vi "Process.vi"(8 "error in":errorcluster, 11 "Instrument.Aerotech":refnum<class "Instrument.Aerotech.lvclass">) -> (0 "error out":errorcluster, 3 "Instrument.Aerotech out":refnum<class "Instrument.Aerotech.lvclass">)   [LabVIEW 2019, in "Instrument.Aerotech.lvclass"]
doc: "---------------------------------------------------------------\nJKI State Machine Objects™\nhttp://jki.net/state-machine-objects/\nCopyright (C) 2005-2015, JKI <info@jki.net>\nALL RIGHTS RESERVED"
uses:
  Instrument.Aerotech.lvclass
  <vilib>/JKI/JKI SMO/SMO/SMO.lvclass
  <vilib>/JKI/JKI SMO/SMO/Typedefs/Parent Call--Enum.ctl
  C:/Program Files (x86)/National Instruments/LabVIEW 2019/user.lib/LevyLab/Instrument Framework/Instrument Types/Delay Line/Instrument.DelayLine.lvclass
  C:/Program Files (x86)/National Instruments/LabVIEW 2019/user.lib/LevyLab/Instrument Framework/Instrument/Instrument.lvclass
  C:/Program Files (x86)/National Instruments/LabVIEW 2019/vi.lib/JKI/JKI SMO/SMO/SMO.lvclass
  <userlib>/LevyLab/Instrument Framework/Instrument Types/Delay Line/Instrument.DelayLine.lvclass
panel:
  # "Example INSTRUMENT"
  # "For instructions on how to use the JKI State Machine Objects, examples and video tutorials, visit:\nhttp://jki.net/state-machine-objects/\n\nJKI State Machine Objects™\nhttp://jki.net/state-machine-objects/\nCopyright (C) 2005-2015, JKI <info@jki.net>\nALL RIGHTS RESERVED"
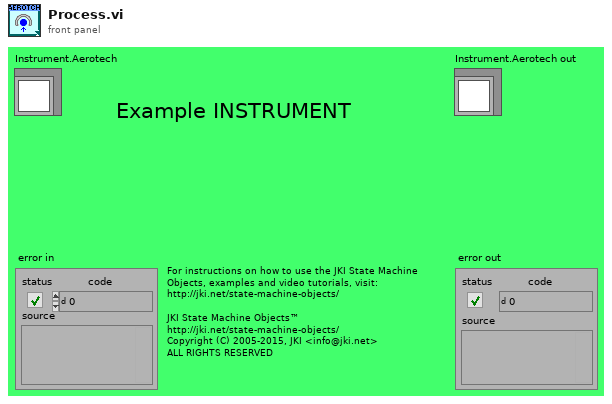
[diagram p1: front panel]
types:
  T1 = typedef "SMO.lvclass/Parent Call--Enum.ctl" = enum16{"Allows parent to run", "Does not request parent to run"}
  T2 = enum32{"invalid app kind", "Development System", "Run Time System", "Student Edition", "Embedded LabVIEW", "Evaluation", "Custom"}
  T3 = enum32{"Invalid", "Standard", "Closed", "Hidden", "Minimized", "Maximized"}
  T4 = enum32{"Bad", "Idle", "Run top level", "Running"}
  T5 = cluster{"Core":cluster{"Current VI Reference":refnum<vi>, "Close Panel on Exit?":bool, "error":errorcluster}, "Self Reference":refnum<class "Instrument.Aerotech.lvclass">}
  T6 = cluster{"Current VI Reference":refnum<vi>, "Close Panel on Exit?":bool, "error":errorcluster}
  T7 = typedef "SMO.lvclass/Protected Events.ctl" = cluster{"StopProcesses":refnum<user-event>, "AbortProcesses":refnum<user-event>, "Config Changed":refnum<user-event>, "Dependency":refnum<user-event>}
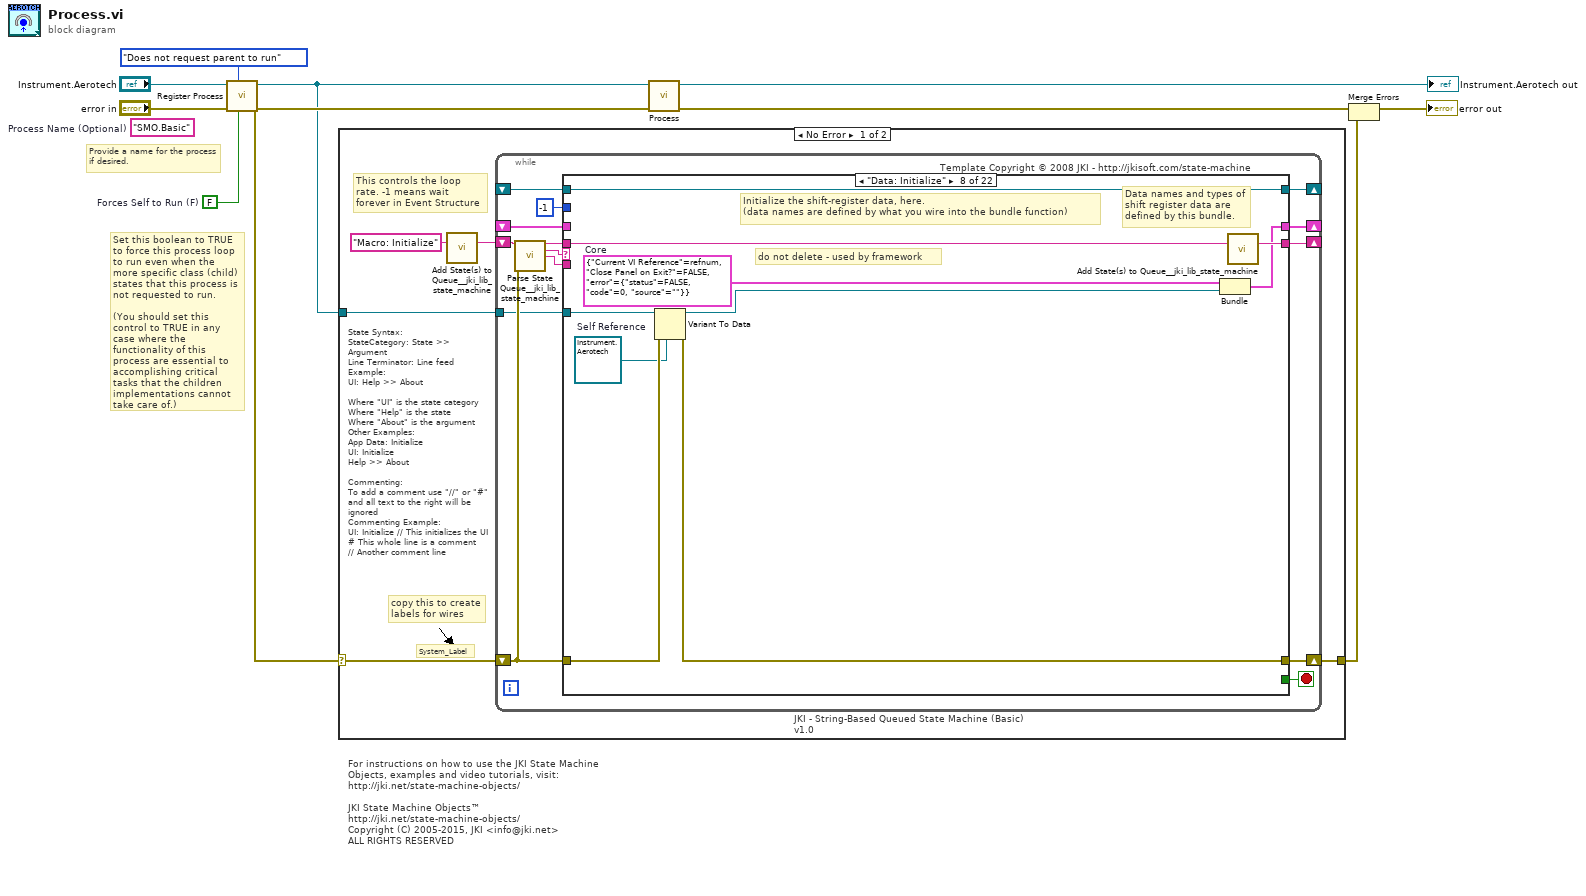
[diagram p0: block diagram]
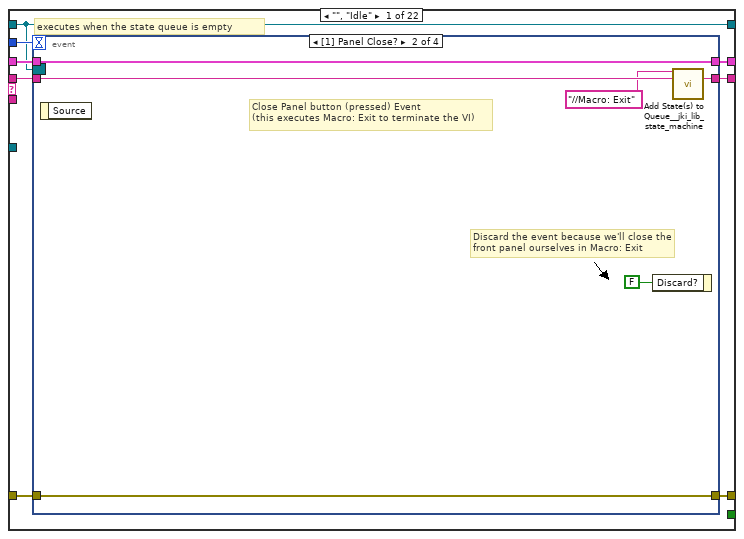
[diagram p2: hidden frame]
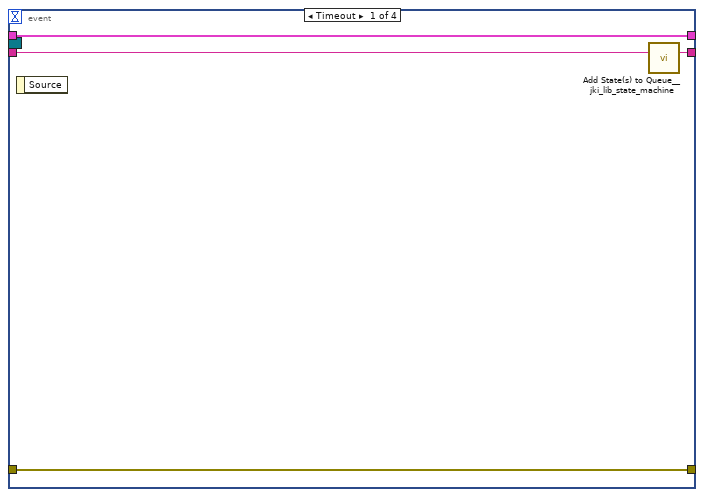
[diagram p3: hidden frame]
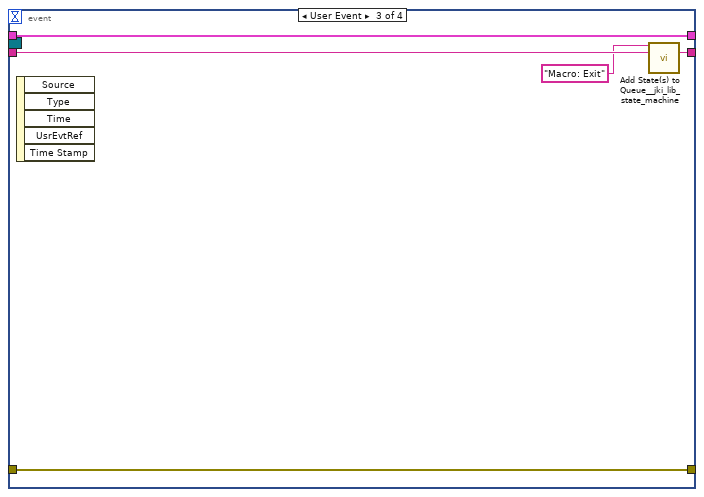
[diagram p4: hidden frame]
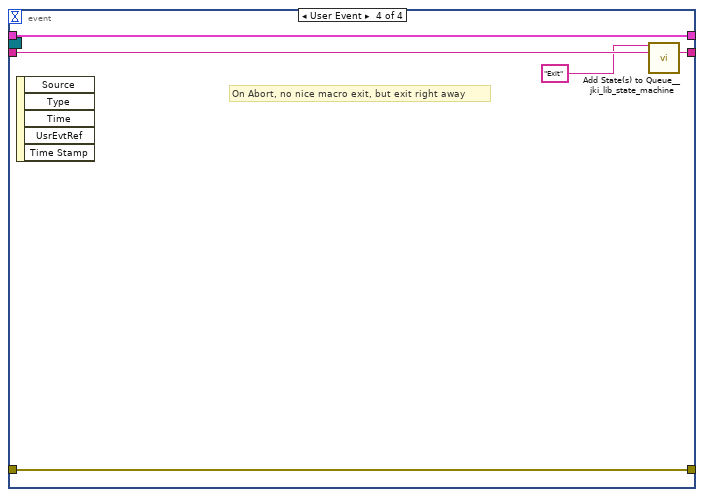
[diagram p5: hidden frame]
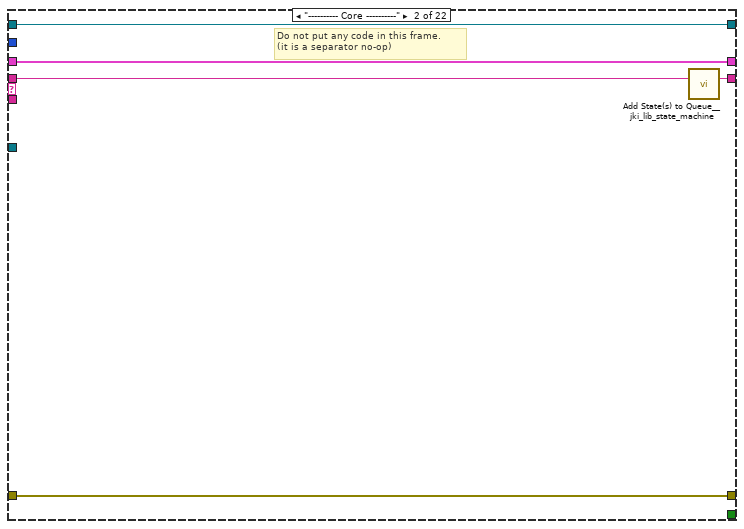
[diagram p6: hidden frame]
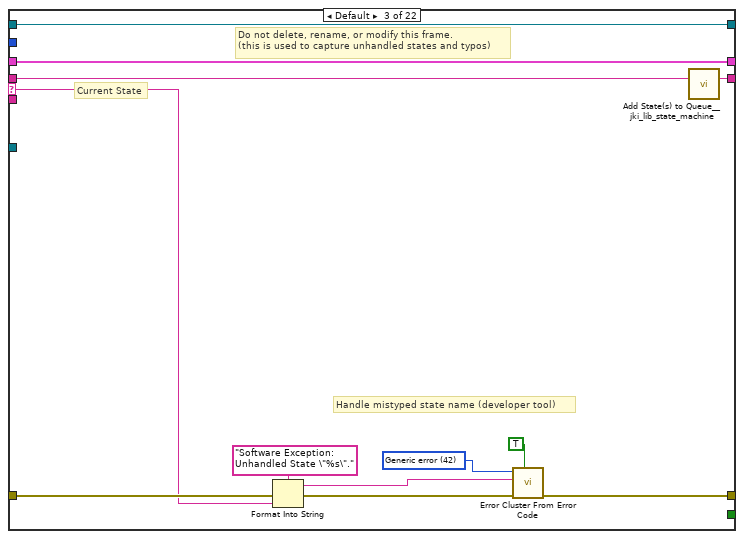
[diagram p7: hidden frame]
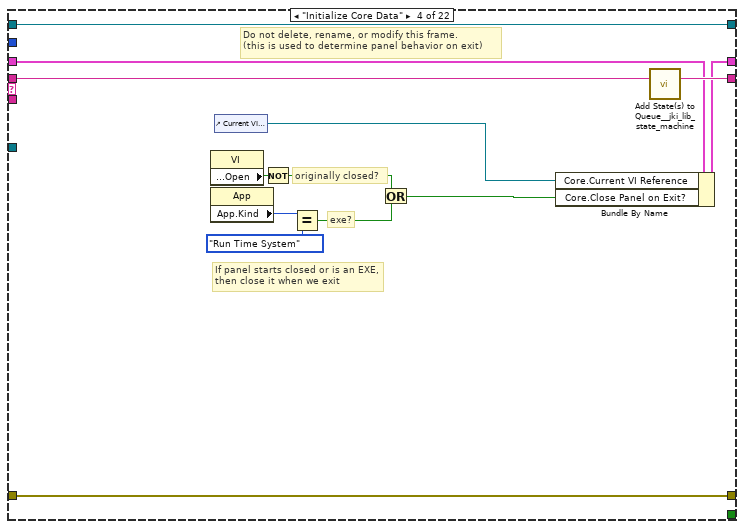
[diagram p8: hidden frame]
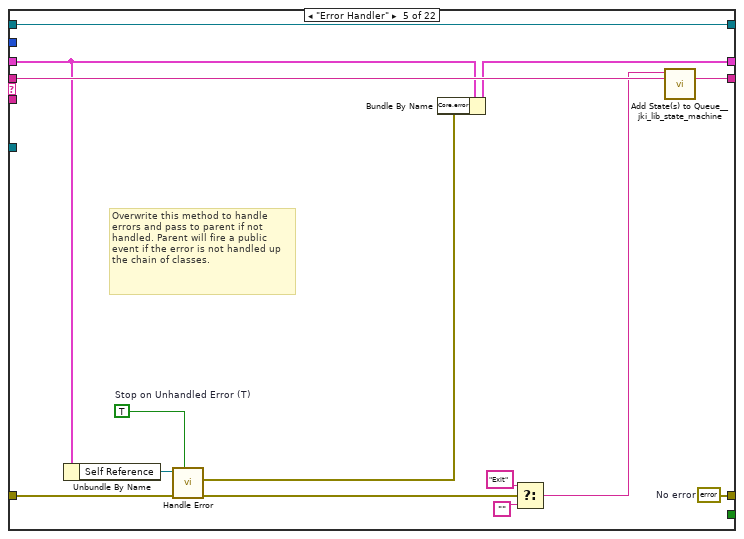
[diagram p9: hidden frame]
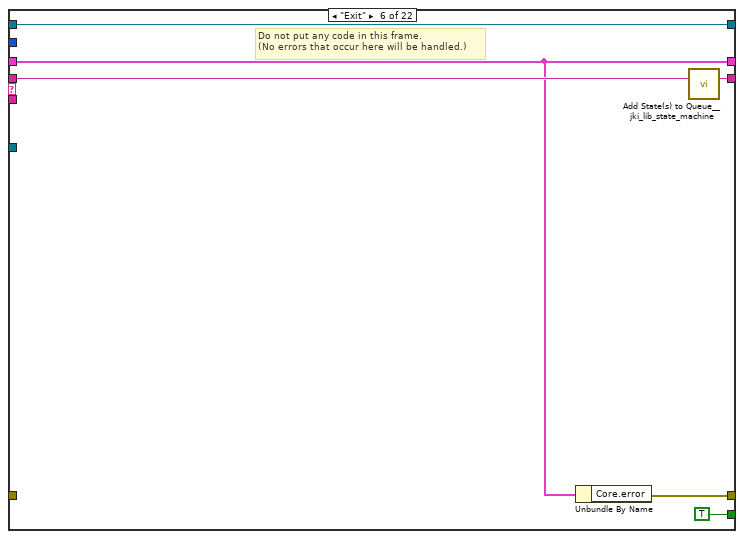
[diagram p10: hidden frame]
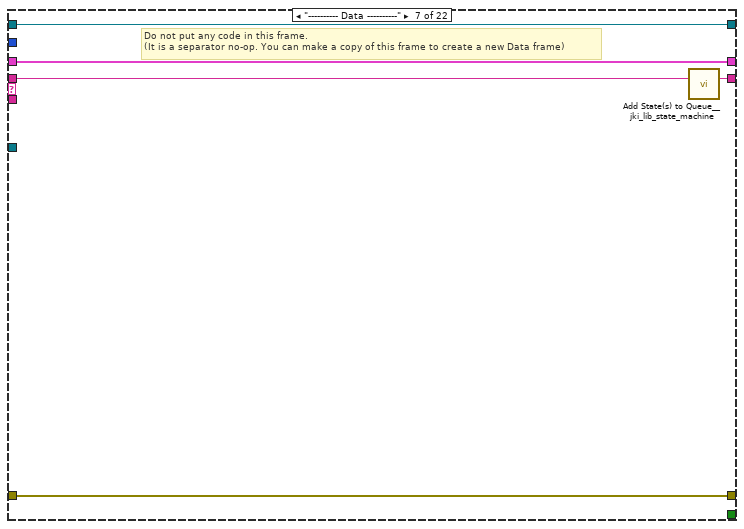
[diagram p11: hidden frame]
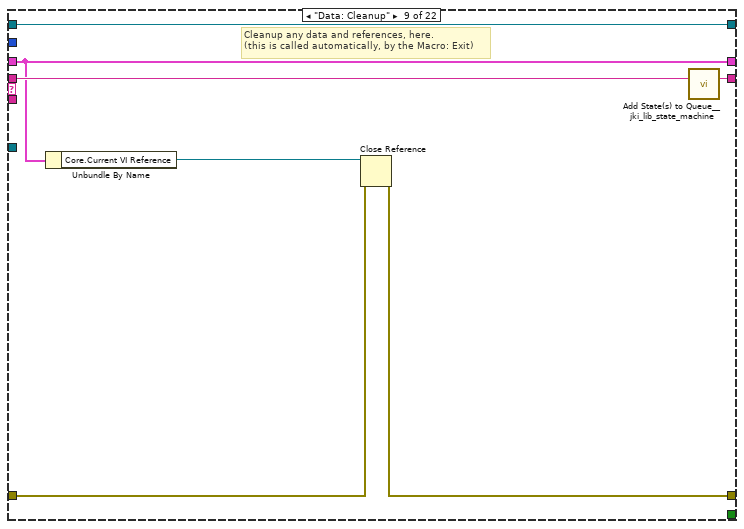
[diagram p12: hidden frame]
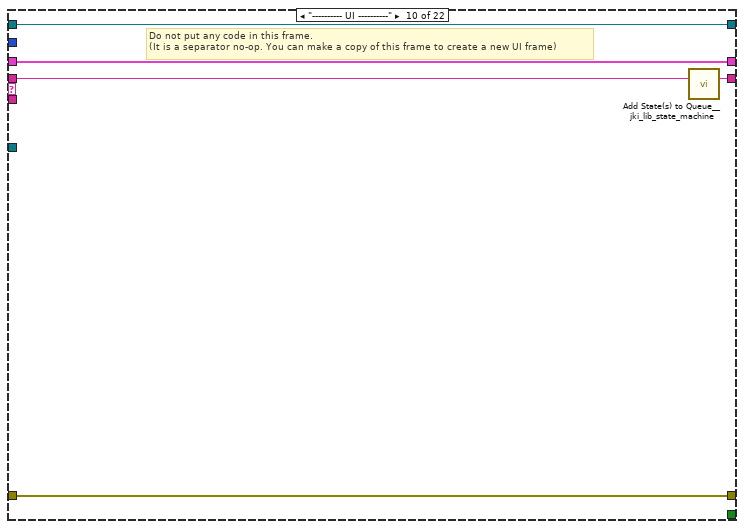
[diagram p13: hidden frame]
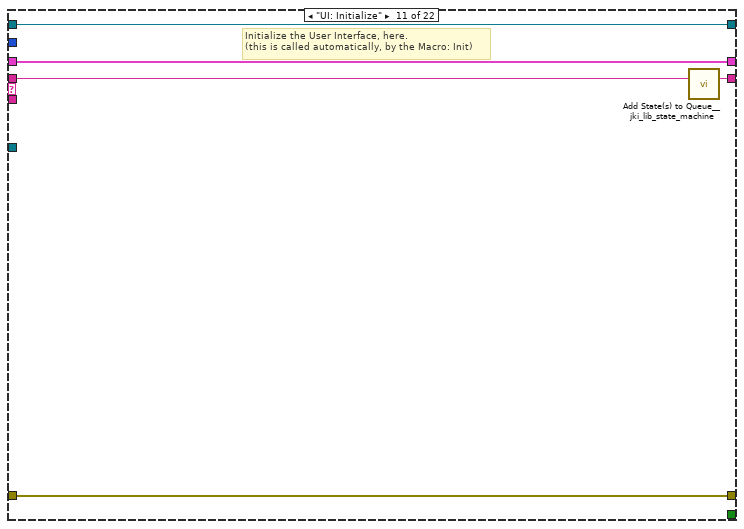
[diagram p14: hidden frame]
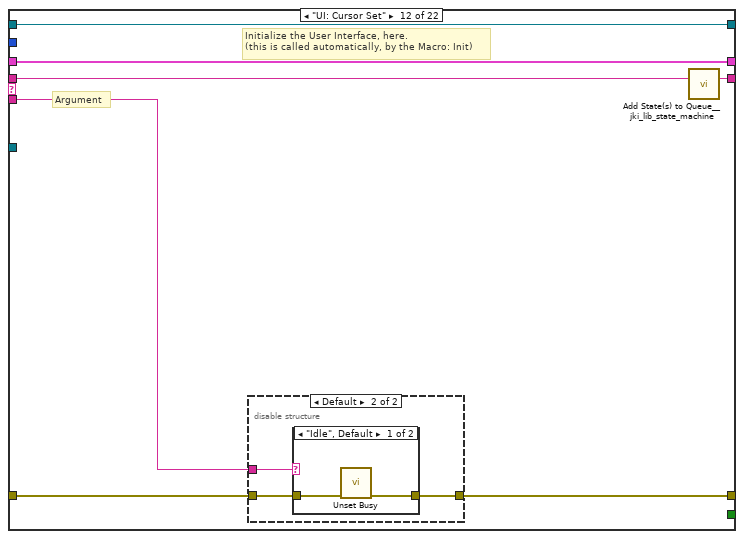
[diagram p15: hidden frame]
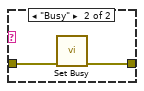
[diagram p17: hidden frame]
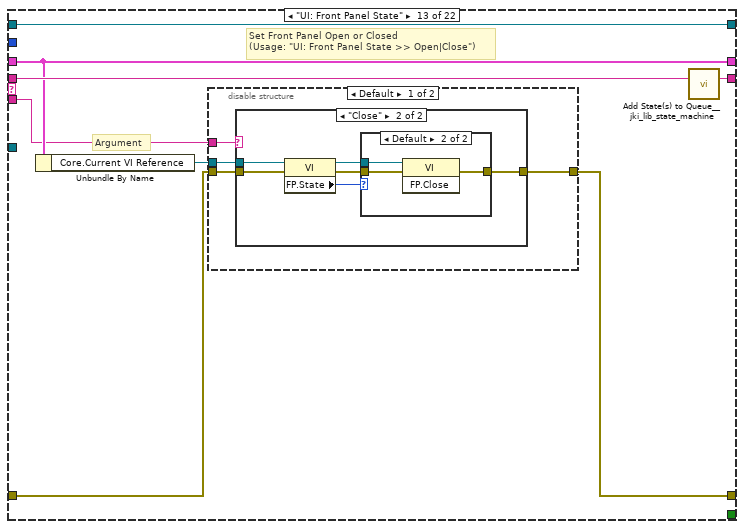
[diagram p18: hidden frame]
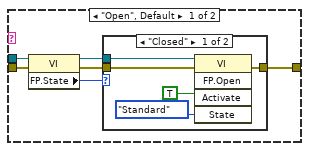
[diagram p19: hidden frame]
diagram:
  w1 = FALSE  # Forces Self to Run (F)
  (unwired) "SMO.Basic"  # Process Name (Optional)
  # "Provide a name for the process\nif desired."
  # "Set this boolean to TRUE to force this process loop to run even when the more specific class (child) states that this process is not requested to run.\n\n(You should set this control to TRUE in any case where the functionality of this process are essential to accomplishing critical tasks that the children implementations cannot take care of.)"
  # "For instructions on how to use the JKI State Machine Objects, examples and video tutorials, visit:\nhttp://jki.net/state-machine-objects/\n\nJKI State Machine Objects™\nhttp://jki.net/state-machine-objects/\nCopyright (C) 2005-2015, JKI <info@jki.net>\nALL RIGHTS RESERVED"
  n1 = call <vilib>:"Register Process.vi"("Forces Self to Run (F)"=w1, "Parent Call"=Parent_Call--Enum."Does not request parent to run", "error in (no error)"="error in", "SMO"="Instrument.Aerotech") -> ("error out"=w7:errorcluster, "SMO out"=w6:refnum<class "Instrument.Aerotech.lvclass">)  [unwired: 6 in]
  n2 = case shown="No Error" w7 {
    selector: w7 -> [w12 w265]
    tunnel: w6 -> [w13 _]
    tunnel: [w11 w265] -> w3
    frame No Error {
      # "State Syntax:\nStateCategory: State >> Argument\nLine Terminator: Line feed\nExample:\nUI: Help >> About\n\nWhere \"UI\" is the state category\nWhere \"Help\" is the state\nWhere \"About\" is the argument\nOther Examples:\nApp Data: Initialize\nUI: Initialize\nHelp >> About\n\nCommenting:\nTo add a comment use \"//\" or \"#\" and all text to the right will be ignored\nCommenting Example:\nUI: Initialize // This initializes the UI\n# This whole line is a comment\n// Another comment line"
      # "copy this to create labels for wires"
      # "This controls the loop rate. -1 means wait forever in Event Structure"
      # "System_Label"
      n3 = call <vilib>:"Add State(s) to Queue__jki_lib_state_machine.vi"("State(s) in (\"\")"="Macro: Initialize") -> ("States Out"=w15:string)  [unwired: 14 in]
      n4 = while "JKI - String-Based Queued State Machine (Basic) v1.0" {
        shift-right: [w22] -> _
        shift-left: _ -> [w21]
        shift-right: [w25] -> w11
        shift-left: w12 -> [w19]
        shift-right: [w24] -> _
        shift-left: w15 -> [w26]
        tunnel: w13 -> [w18]
        shift-right: [w17] -> _
        shift-left: _ -> [w16]
        stop <- w23 stop-if-true
        # "Template Copyright © 2008 JKI - http://jkisoft.com/state-machine"
        n5 = call <vilib>:"Parse State Queue__jki_lib_state_machine.vi"("State Queue"=w26, "Error In (no error)"=w19) -> ("Remaining States"=w28:string, "Current State"=w29:string, "Arguments"=w27:string)  [unwired: 11 in]
        n6 = case shown="\"Data: Initialize\"" w29 {
          selector: w29 -> [_ _ w64 _ _ _ _ _ _ _ _ _ _ _ _ _ _ _ _ _ _ _]
          tunnel: w28 -> [w37 w62 w68 w87 w101 w107 w112 w122 w129 w134 w139 w146 w162 w194 w208 w222 w227 w238 w243 w253 w259 w264]
          tunnel: w27 -> [_ _ _ _ _ _ _ _ _ _ _ w140 w156 _ _ _ _ _ _ _ _ _]
          tunnel: w21 -> [w35 w59 w66 w78 w95 w103 w109 _ w124 w131 w137 w144 w158 w191 w204 w213 w224 w235 w240 w244 w257 w262]
          tunnel: [w34 w60 w70 w84 w96 w102 w110 w118 w125 w132 w136 w141 w159 w192 w206 w220 w225 w229 w241 w248 w255 w260] -> w25
          tunnel: w19 -> [w33 w60 w69 w84 w97 _ w110 w119 w126 w132 w136 w142 w160 w192 w206 w220 w225 w230 w241 w249 w255 w260]
          tunnel: [w36 w61 w67 w86 w100 w106 w111 w121 w128 w133 w138 w145 w161 w193 w207 w221 w226 w237 w242 w252 w258 w263] -> w24
          tunnel: [_ _ _ _ _ TRUE _ _ _ _ _ _ _ _ _ _ _ _ _ _ _ _] -> w23
          tunnel: [w32 w59 w66 w85 w94 w103 w109 w120 w124 w131 w137 w144 w158 w191 w204 w213 w224 w235 w240 w244 w257 w262] -> w22
          tunnel: -1 ("Timeout") -> [w31 _ _ _ _ _ _ _ _ _ _ _ _ _ _ _ _ _ _ _ _ _]
          tunnel: w18 -> [_ _ _ _ _ _ _ w116 _ _ _ _ _ _ _ _ _ _ _ _ _ _]
          tunnel: [w30 w58 w63 w75 w99 w104 w108 w115 w123 w130 w135 w143 w155 w190 w205 w214 w223 w236 w239 w251 w256 w261] -> w17
          tunnel: w16 -> [w30 w58 w63 w75 w99 w104 w108 w115 w123 w130 w135 w143 w155 w190 w205 w214 w223 w236 w239 _ w256 w261]
          frame "", "Idle" {
            # "executes when the state queue is empty"
            n7 = event shown="[1] Panel Close?" {
              selector: w30 -> [_ _ _ _]
              dyn-events: _ -> [_ _ _ _]
              timeout: w31 -> [_ _ _ _]
              tunnel: w37 -> [w41 w47 w52 w57]
              tunnel: [w40 w46 w51 w56] -> w36
              tunnel: w35 -> [w38 w44 w49 w54]
              tunnel: [w39 w45 w50 w55] -> w34
              tunnel: w33 -> [w39 w45 w50 w55]
              tunnel: [w38 w44 w49 w54] -> w32
              event Timeout {
                n8 = event-data() -> ()  [unwired: 1 in, 1 out]
                n9 = call <vilib>:"Add State(s) to Queue__jki_lib_state_machine.vi"("State(s) in (\"\")"=w41) -> ("States Out"=w40:string)  [unwired: 14 in]
              }
              event Panel Close? {
                # "Discard the event because we'll close the front panel ourselves in Macro: Exit"
                # "Close Panel button (pressed) Event\n(this executes Macro: Exit to terminate the VI)"
                n10 = event-data() -> ()  [unwired: 1 in, 1 out]
                n11 = event-data("Discard?"=FALSE) -> ()  [unwired: 1 in, 1 out]
                n12 = call <vilib>:"Add State(s) to Queue__jki_lib_state_machine.vi"("State(s) in Front (\"\")"="//Macro: Exit", "State(s) in (\"\")"=w47) -> ("States Out"=w46:string)  [unwired: 13 in]
              }
              event User Event {
                n13 = event-data() -> ()  [unwired: 1 in, 5 out]
                n14 = call <vilib>:"Add State(s) to Queue__jki_lib_state_machine.vi"("State(s) in Front (\"\")"="Macro: Exit", "State(s) in (\"\")"=w52) -> ("States Out"=w51:string)  [unwired: 13 in]
              }
              event User Event {
                # "On Abort, no nice macro exit, but exit right away"
                n15 = event-data() -> ()  [unwired: 1 in, 5 out]
                n16 = call <vilib>:"Add State(s) to Queue__jki_lib_state_machine.vi"("State(s) in Front (\"\")"="Exit", "State(s) in (\"\")"=w57) -> ("States Out"=w56:string)  [unwired: 13 in]
              }
            }
          }
          frame "---------- Core ----------" {
            # "Do not put any code in this frame.\n(it is a separator no-op)"
            n17 = call <vilib>:"Add State(s) to Queue__jki_lib_state_machine.vi"("State(s) in (\"\")"=w62) -> ("States Out"=w61:string)  [unwired: 14 in]
          }
          frame Default {
            w73 = 42 items=["No error", "Argument error", "Memory is full", "Out of zone", "End of file", "File already open", "Generic file I/O error", "File not found", "File permission error", "Disk is full", "Duplicate path", "Too many files open", "System feature not enabled", "Resource file not found", "Cannot add resource", "Resource not found", "Image not found", "Image memory error", "Pen does not exist", "Config type invalid", "Config token not found", "Config parse error", "Config memory error", "Bad external code format", "Bad external code offset", "External code not present", "Null window", "Destroy window error", "Null menu", "Print aborted", "Bad print record", "Print driver error", "Windows error during printing", "Memory error during printing", "Print dialog error", "Generic print error", "Invalid device refnum", "Device not found", "Device parameter error", "Device unit error", "Cannot open device", "Device call aborted", "Generic error", "Cancelled by user", "Object ID too low", "Object ID too high", "Object not in heap", "Unknown heap", "Unknown object (invalid DefProc)", "Unknown object (DefProc not in table)", "Message out of range", "Invalid (null) method", "Unknown message", "Manager call not supported", "Bad address", "Network operation in progress", "Network operation timed out", "Connection is busy", "Network attribute not supported", "Network error", "Address in use", "System out of memory", "Connection aborted", "Connection refused", "Not connected", "Already connected", "Connection closed", "Initialization error (interapplication manager)", "Bad occurrence", "Wait on unbound occurrence handler", "Occurrence queue overflow", "Datalog type conflict", "Unused", "Unrecognized type (interapplication manager)", "Memory corrupt", "Failed to make temporary DLL", "Old CIN version", "Drag socket not found", "Failed to load drop-object", "Failed to register OLE object", "Failed to release OLE object", "Format specifier type mismatch", "Unknown format specifier", "Too few format specifiers", "Too many format specifiers", "Scan failed", "Newer CIN version", "Error converting to variant", "Runtime menu error", "Password tampered", "Variant attribute not found", "Incompatible variant data type", "Event data is not available", "Event Store is not present", "Occurrence is not found", "Event Queue is not created", "Event info is not available", "Refnum passed is NULL", "Error retrieving Class GUID", "Error retrieving CoClass GUID", "Error retrieving TypeLib GUID.", "Bad built application magic bytes.", "Specific driver is different from the specific driver associated with the Logical Name.", "There is no session opened to the class driver.", "Max Error", "MAX - Error with config objects", "MAX - Error loading configuration", "MAX - Group not supported"]
            # "Current State"
            # "Do not delete, rename, or modify this frame.\n(this is used to capture unhandled states and typos)"
            # "Handle mistyped state name (developer tool)"
            n18 = Format Into String(format string="Software Exception: Unhandled State \"%s\"." ("message"), error in=w69, w64) -> (resulting string=w72:string, error out=w71:errorcluster)  [unwired: 1 in]
            n19 = call <vilib>:"Error Cluster From Error Code.vi"("show call chain? (False)"=TRUE, "error in (no error)"=w71, "error message (\"\")"=w72, "error code (0)"=w73) -> ("error out"=w70:errorcluster)  [unwired: 5 in]
            n20 = call <vilib>:"Add State(s) to Queue__jki_lib_state_machine.vi"("State(s) in (\"\")"=w68) -> ("States Out"=w67:string)  [unwired: 14 in]
          }
          frame "Initialize Core Data" {
            # "Do not delete, rename, or modify this frame.\n(this is used to determine panel behavior on exit)"
            # "originally closed?"
            # "exe?"
            # "If panel starts closed or is an EXE, then close it when we exit"
            n21 = property class="VI"() -> ("Front Panel.Open"=w83:bool)  [unwired: 2 in, 2 out]
            n22 = property class="App"() -> ("App.Kind"=w82:T2)  [unwired: 2 in, 2 out]
            n23 = control-ref of="Current VI Reference"() -> (w76:refnum<vi>)
            n24 = Not(x=w83) -> (.not. x?=w80:bool)
            n25 = Equal?(x=w82, y=T2."Run Time System" ("Application:Kind")) -> (x = y?=w79:bool)
            n26 = Or(x=w80, y=w79) -> (x .or. y?=w77:bool)
            n27 = Bundle By Name(cluster=w78, "Core.Current VI Reference"=w76, "Core.Close Panel on Exit?"=w77) -> (w85:T5)
            n28 = call <vilib>:"Add State(s) to Queue__jki_lib_state_machine.vi"("State(s) in (\"\")"=w87) -> ("States Out"=w86:string)  [unwired: 14 in]
          }
          frame "Error Handler" {
            w88 = TRUE  # Stop on Unhandled Error (T)
            w96 = errorcluster {"status"=FALSE, "code"=0, "source"=""}  # No error
            # "Overwrite this method to handle errors and pass to parent if not handled. Parent will fire a public event if the error is not handled up the chain of classes."
            n29 = Unbundle By Name(w95) -> ("Self Reference"=w98:refnum<class "Instrument.Aerotech.lvclass">)
            n30 = call-dynamic "Handle Error.vi"("Stop on Unhandled Error (T)"=w88, "error in"=w97, "SMO"=w98) -> ("handling error"=w89:errorcluster, "Unhandled error"=w92:errorcluster)  [unwired: 6 in, 1 out]
            n31 = Bundle By Name(cluster=w95, "Core.error"=w92) -> (w94:T5)
            n32 = Select(t="Exit", s=w89, f="") -> (s? t:f=w93:string)
            n33 = call <vilib>:"Add State(s) to Queue__jki_lib_state_machine.vi"("State(s) in Front (\"\")"=w93, "State(s) in (\"\")"=w101) -> ("States Out"=w100:string)  [unwired: 13 in]
          }
          frame "Exit" {
            # "Do not put any code in this frame.\n(No errors that occur here will be handled.)"
            n34 = Unbundle By Name(w103) -> ("Core.error"=w102:errorcluster)
            n35 = call <vilib>:"Add State(s) to Queue__jki_lib_state_machine.vi"("State(s) in (\"\")"=w107) -> ("States Out"=w106:string)  [unwired: 14 in]
          }
          frame "---------- Data ----------" {
            # "Do not put any code in this frame.\n(It is a separator no-op. You can make a copy of this frame to create a new Data frame)"
            n36 = call <vilib>:"Add State(s) to Queue__jki_lib_state_machine.vi"("State(s) in (\"\")"=w112) -> ("States Out"=w111:string)  [unwired: 14 in]
          }
          frame "Data: Initialize" {
            w114 = T6 {"Current VI Reference"=refnum, "Close Panel on Exit?"=FALSE, "error"={"status"=FALSE, "code"=0, "source"=""}}  # Core
            w117 = refnum<class "Instrument.Aerotech.lvclass"> refnum  # Self Reference
            # "do not delete - used by framework"
            # "Data names and types of shift register data are defined by this bundle."
            # "Initialize the shift-register data, here.\n(data names are defined by what you wire into the bundle function)"
            n37 = Variant To Data(error in=w119, type=w117, Variant=w116) -> (data=w113:refnum<class "Instrument.Aerotech.lvclass">, error out=w118:errorcluster)
            n38 = Bundle("Core"=w114, "Self Reference"=w113) -> (w120:T5)  [unwired: 1 in]
            n39 = call <vilib>:"Add State(s) to Queue__jki_lib_state_machine.vi"("State(s) in (\"\")"=w122) -> ("States Out"=w121:string)  [unwired: 14 in]
          }
          frame "Data: Cleanup" {
            # "Cleanup any data and references, here.\n(this is called automatically, by the Macro: Exit)"
            n40 = Unbundle By Name(w124) -> ("Core.Current VI Reference"=w127:refnum<vi>)
            n41 = Close Reference(reference=w127, error in (no error)=w126) -> (error out=w125:errorcluster)
            n42 = call <vilib>:"Add State(s) to Queue__jki_lib_state_machine.vi"("State(s) in (\"\")"=w129) -> ("States Out"=w128:string)  [unwired: 14 in]
          }
          frame "---------- UI ----------" {
            # "Do not put any code in this frame.\n(It is a separator no-op. You can make a copy of this frame to create a new UI frame)"
            n43 = call <vilib>:"Add State(s) to Queue__jki_lib_state_machine.vi"("State(s) in (\"\")"=w134) -> ("States Out"=w133:string)  [unwired: 14 in]
          }
          frame "UI: Initialize" {
            # "Initialize the User Interface, here.\n(this is called automatically, by the Macro: Init)"
            n44 = call <vilib>:"Add State(s) to Queue__jki_lib_state_machine.vi"("State(s) in (\"\")"=w139) -> ("States Out"=w138:string)  [unwired: 14 in]
          }
          frame "UI: Cursor Set" {
            # "Argument"
            # "Initialize the User Interface, here.\n(this is called automatically, by the Macro: Init)"
            n45 = disable-structure shown="Default" {
              disable-tunnel: w142 -> [w147 w150]
              disable-tunnel: [w147 w149] -> w141
              disable-tunnel: w140 -> [_ w148]
              frame condition #0 {
              }
              frame condition #1 (active) {
                n46 = case shown="\"Idle\", Default" w148 {
                  tunnel: w150 -> [w152 w154]
                  tunnel: [w151 w153] -> w149
                  frame "Idle", Default {
                    n47 = call <vilib>:"Unset Busy.vi"("error in (no error)"=w152) -> ("error out"=w151:errorcluster)  [unwired: 10 in]
                  }
                  frame "Busy" {
                    n48 = call <vilib>:"Set Busy.vi"("error in (no error)"=w154) -> ("error out"=w153:errorcluster)  [unwired: 9 in, 1 out]
                  }
                }
              }
            }
            n49 = call <vilib>:"Add State(s) to Queue__jki_lib_state_machine.vi"("State(s) in (\"\")"=w146) -> ("States Out"=w145:string)  [unwired: 14 in]
          }
          frame "UI: Front Panel State" {
            # "Argument"
            # "Set Front Panel Open or Closed\n(Usage: \"UI: Front Panel State >> Open|Close\")"
            n50 = Unbundle By Name(w158) -> ("Core.Current VI Reference"=w157:refnum<vi>)
            n51 = disable-structure shown="Default" {
              disable-tunnel: w160 -> [w166 w189]
              disable-tunnel: [w165 w189] -> w159
              disable-tunnel: w157 -> [w164 _]
              disable-tunnel: w156 -> [w163 _]
              frame condition #0 (active) {
                n52 = case shown="\"Close\"" w163 {
                  tunnel: w166 -> [w170 w183]
                  tunnel: [w172 w184] -> w165
                  tunnel: w164 -> [w171 w181]
                  frame "Open", Default {
                    n53 = property class="VI"(reference=w171, error in=w170) -> (reference out=w168:refnum<vi>, error out=w169:errorcluster, "FP.State"=w167:T3)
                    n54 = case shown="\"Closed\"" w167 {
                      tunnel: [w175 w178] -> w172
                      tunnel: w169 -> [w174 w178]
                      tunnel: w168 -> [w173 _]
                      frame "Closed" {
                        n55 = invoke class="VI" method="FP.Open"(reference=w173, error in=w174, "Activate"=TRUE, "State"=T3."Standard") -> (error out=w175:errorcluster)  [unwired: 1 in, 4 out]
                      }
                      frame Default {
                      }
                    }
                  }
                  frame "Close" {
                    n56 = property class="VI"(reference=w181, error in=w183) -> (reference out=w180:refnum<vi>, error out=w182:errorcluster, "FP.State"=w179:T3)
                    n57 = case shown="Default" w179 {
                      tunnel: [w185 w188] -> w184
                      tunnel: w182 -> [w185 w187]
                      tunnel: w180 -> [_ w186]
                      frame "Invalid", "Closed" {
                      }
                      frame Default {
                        n58 = invoke class="VI" method="FP.Close"(reference=w186, error in=w187) -> (error out=w188:errorcluster)  [unwired: 1 in, 2 out]
                      }
                    }
                  }
                }
              }
              frame condition #1 {
              }
            }
            n59 = call <vilib>:"Add State(s) to Queue__jki_lib_state_machine.vi"("State(s) in (\"\")"=w162) -> ("States Out"=w161:string)  [unwired: 14 in]
          }
          frame "---------- Macro ----------" {
            # "Do not put any code in this frame.\n(It is a separator no-op. You can make a copy of this frame to create a new Macro frame)"
            n60 = call <vilib>:"Add State(s) to Queue__jki_lib_state_machine.vi"("State(s) in (\"\")"=w194) -> ("States Out"=w193:string)  [unwired: 14 in]
          }
          frame "Macro: Initialize" {
            w199 = "UI: Initialize\nUI: Front Panel State >> Open"  # UI: Initialize UI: Front Panel State >> Open
            w195 = "Process: Sync"
            # "Initialization Macro\n(This is called once, when the VI starts)"
            n61 = control-ref of="This VI"() -> (w197:refnum<vi>)
            n62 = property class="VI"(reference=w197) -> ("Exec.State"=w196:T4)  [unwired: 1 in, 2 out]
            n63 = Equal?(x=w196, y=T4."Run top level") -> (x = y?=w202:bool)
            n64 = Select(t=w195, s=w202, f="") -> ()  [unwired: 1 out]
            n65 = call <vilib>:"Add State(s) to Queue__jki_lib_state_machine.vi"("State(s) in Front (\"\")"="Data: Initialize\nInitialize Core Data\nEvents: Register", "State(s) in (\"\")"=w195, "State(s) at Back (\"\")"=w199) -> ("States Out"=w198:string)  [unwired: 12 in]
            n66 = call <vilib>:"Add State(s) to Queue__jki_lib_state_machine.vi"("State(s) in Front (\"\")"=w198, "State(s) in (\"\")"=w208) -> ("States Out"=w207:string)  [unwired: 13 in]
          }
          frame "Macro: Exit" {
            # "Exit Macro\n(This is called once, when the VI exits)"
            n67 = Unbundle By Name(w213) -> ("Core.Close Panel on Exit?"=w219:bool)
            n68 = Select(t="UI: Front Panel State >> Close", s=w219, f="") -> (s? t:f=w216:string)
            n69 = call <vilib>:"Add State(s) to Queue__jki_lib_state_machine.vi"("State(s) in Front (\"\")"="Data: Cleanup\nEvents: Unregister", "State(s) in (\"\")"="Process: Sync", "State(s) at Back (\"\")"="Exit") -> ("States Out"=w210:string)  [unwired: 12 in]
            n70 = call <vilib>:"Add State(s) to Queue__jki_lib_state_machine.vi"("State(s) in (\"\")"=w216, "State(s) at Back (\"\")"=w210) -> ("States Out"=w215:string)  [unwired: 13 in]
            n71 = call <vilib>:"Add State(s) to Queue__jki_lib_state_machine.vi"("State(s) in Front (\"\")"=w215, "State(s) in (\"\")"=w222) -> ("States Out"=w221:string)  [unwired: 13 in]
          }
          frame "---------- Process ----------" {
            # "Template Separator\n(You can make a copy of, or modify, this frame)"
            n72 = call <vilib>:"Add State(s) to Queue__jki_lib_state_machine.vi"("State(s) in (\"\")"=w227) -> ("States Out"=w226:string)  [unwired: 14 in]
          }
          frame "Process: Sync" {
            n73 = Unbundle By Name(w235) -> ("Self Reference"=w231:refnum<class "Instrument.Aerotech.lvclass">)
            n74 = call <vilib>:"WaitOnProcessSync.vi"("error in (no error)"=w230, "SMO"=w231) -> ("error out"=w229:errorcluster, "Don't run?"=w234:bool)  [unwired: 7 in, 1 out]
            n75 = Select(t="Data: Cleanup\nEvents: Unregister\nExit", s=w234, f="") -> (s? t:f=w228:string)
            n76 = call <vilib>:"Add State(s) to Queue__jki_lib_state_machine.vi"("State(s) in Front (\"\")"=w228, "State(s) in (\"\")"=w238) -> ("States Out"=w237:string)  [unwired: 13 in]
          }
          frame "---------- Events ----------" {
            # "Template Separator\n(You can make a copy of, or modify, this frame)"
            n77 = call <vilib>:"Add State(s) to Queue__jki_lib_state_machine.vi"("State(s) in (\"\")"=w243) -> ("States Out"=w242:string)  [unwired: 14 in]
          }
          frame "Events: Register" {
            # "Expand to add\nmore events"
            n78 = Unbundle By Name(w244) -> ("Self Reference"=w245:refnum<class "Instrument.Aerotech.lvclass">)
            n79 = call <vilib>:"GetProtectedEvents.vi"("SMO"=w245) -> ("error out"=w246:errorcluster, "SMO Protected Events"=w250:T7)  [unwired: 8 in, 1 out]
            n80 = register-events(w250) -> (reference out=w251:refnum<event-registration>, error out=w247:errorcluster)  [unwired: 2 in]
            n81 = Merge Errors(w249, w247, w246) -> (w248:errorcluster)
            n82 = call <vilib>:"Add State(s) to Queue__jki_lib_state_machine.vi"("State(s) in (\"\")"=w253) -> ("States Out"=w252:string)  [unwired: 14 in]
          }
          frame "Events: Unregister" {
            n83 = Unregister For Events(event registration refnum=w256, error in=w255) -> (error out=w254:errorcluster)
            n84 = call <vilib>:"Clear Errors.vi"("error in (no error)"=w254) -> ()  [unwired: 5 in, 2 out]
            n85 = call <vilib>:"Add State(s) to Queue__jki_lib_state_machine.vi"("State(s) in (\"\")"=w259) -> ("States Out"=w258:string)  [unwired: 14 in]
          }
          frame "---------- Action ----------" {
            n86 = call <vilib>:"Add State(s) to Queue__jki_lib_state_machine.vi"("State(s) in (\"\")"=w264) -> ("States Out"=w263:string)  [unwired: 14 in]
          }
        }
      }
    }
    frame Error {
    }
  }
  n87 = call-parent "Process.vi"("error in"=w7, "Instrument"=w6) -> ("error out"=w4:errorcluster, "Instrument out"=→"Instrument.Aerotech out":refnum<class "Instrument.Aerotech.lvclass">)  [unwired: 8 in]
  n88 = Merge Errors(w4, w3) -> (→"error out":errorcluster)
